vi "Exit Multi Frame Structure.vi"(0 "Diagram in":refnum<vi>, 5 "Outputs":refnum<vi>[][](array[refnum]), 11 "error in (no error)":errorcluster) -> (4 "Diagram out":refnum<vi>, 6 "Outputs":refnum<vi>[](array[refnum]), 15 "error out":errorcluster)   [LabVIEW 2015, in "Scripting.lvlib"]
doc: "Exits the Multi Frame Structure that owns <B>Diagram in</B>, supplying the structure's owning diagram at <B>Diagram out</B>."
uses:
  Scripting.lvlib
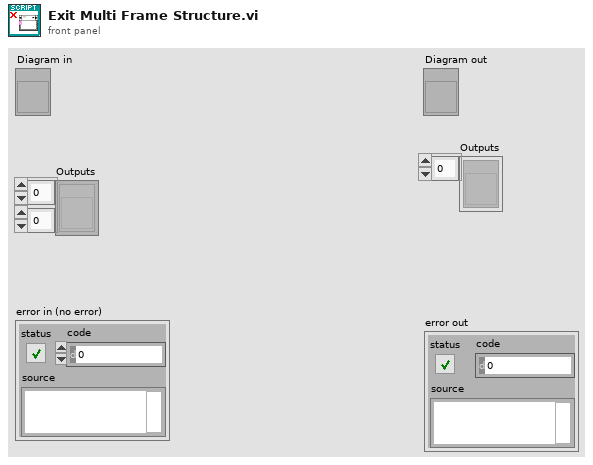
[diagram p1: front panel]
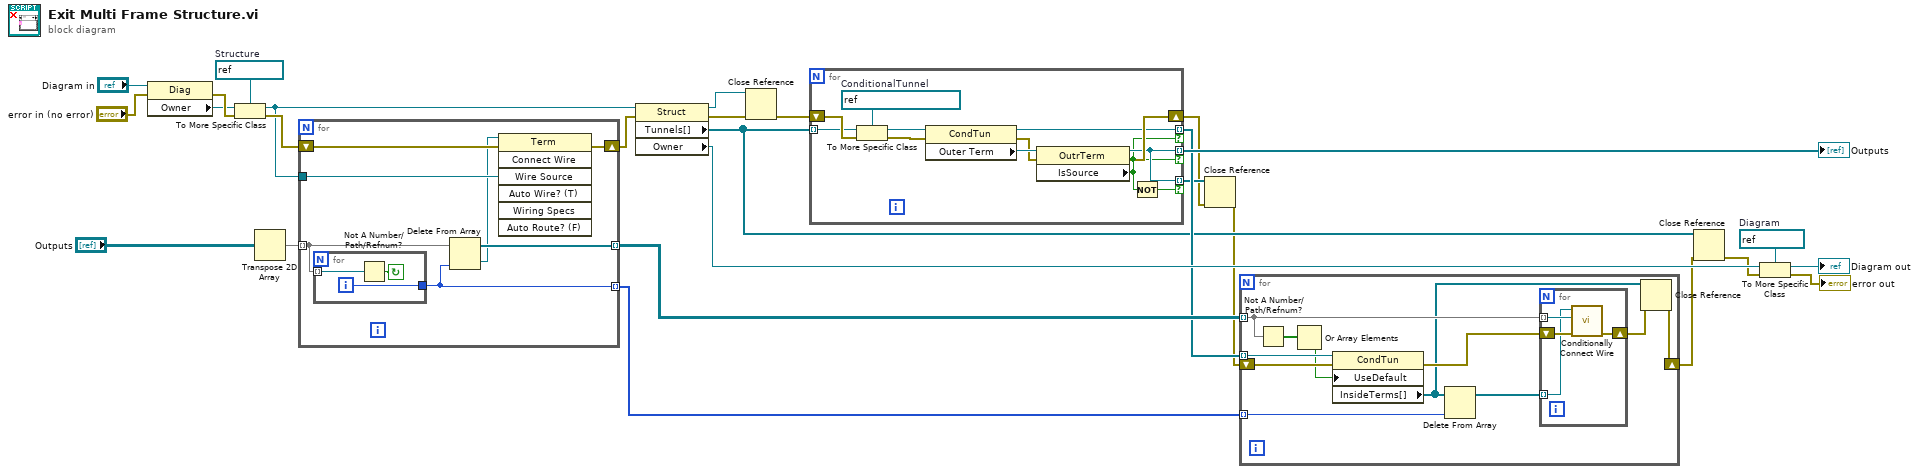
[diagram p0: block diagram]
diagram:
  w23 = refnum<vi> refnum  # Diagram
  w25 = refnum<vi> refnum  # Structure
  n1 = property class="Diag"(reference="Diagram in", error in="error in (no error)") -> (error out=w26:errorcluster, "Owner"=w24:refnum<vi>)  [unwired: 1 out]
  n2 = To More Specific Class(target class=w25, reference=w24, error in=w26) -> (specific class reference=w21:refnum<vi>, error out=w27:errorcluster)
  n3 = Transpose 2D Array(2D array="Outputs") -> (transposed array=w13:refnum<vi>[][])
  n4 = for {
    tunnel: w21 -> [w33]
    shift-right: [w32] -> w20
    shift-left: w27 -> [w34]
    tunnel: w13 -> [w28] mode=indexing
    tunnel: [w31] -> w19 mode=indexing
    tunnel: [w29] -> w9 mode=indexing
    n5 = for {
      tunnel: w28 -> [w35] mode=indexing
      tunnel: [w36] -> w29
      i -> [w36]
      stop <- w37 continue-if-true
      n6 = Not A Number/Path/Refnum?(number/path/refnum=w35) -> (NaN/Path/Refnum?=w37:bool)
    }
    n7 = Delete From Array(array=w28, index=w29) -> (deleted portion=w30:refnum<vi>, array with subset deleted=w31:refnum<vi>[])  [unwired: 1 in]
    n8 = invoke class="Term" method="Connect Wire"(reference=w30, error in=w34, "Wire Source"=w33) -> (error out=w32:errorcluster)  [unwired: 4 in, 6 out]
  }
  n9 = property class="Struct"(reference=w21, error in=w20) -> (reference out=w7:refnum<vi>, error out=w12:errorcluster, "Tunnels[]"=w6:refnum<vi>[], "Owner"=w22:refnum<vi>)
  n10 = Close Reference(reference=w7, error in (no error)=w12) -> (error out=w8:errorcluster)
  n11 = for {
    tunnel: w6 -> [w43] mode=indexing
    tunnel: [w40] -> w15 mode=indexing if=w38
    shift-right: [w46] -> w2
    shift-left: w8 -> [w49]
    tunnel: [w45] -> w14 mode=indexing if=w38
    tunnel: [w40] -> w3 mode=indexing if=w39
    w41 = refnum<vi> refnum  # ConditionalTunnel
    n12 = To More Specific Class(target class=w41, reference=w43, error in=w49) -> (specific class reference=w42:refnum<vi>, error out=w44:errorcluster)
    n13 = property class="CondTun"(reference=w42, error in=w44) -> (reference out=w45:refnum<vi>, error out=w47:errorcluster, "Outer Term"=w48:refnum<vi>)
    n14 = property class="OutrTerm"(reference=w48, error in=w47) -> (reference out=w40:refnum<vi>, error out=w46:errorcluster, "IsSource"=w38:bool)
    n15 = Not(x=w38) -> (.not. x?=w39:bool)
  }
  "Outputs" <- w15
  n16 = Close Reference(reference=w3, error in (no error)=w2) -> (error out=w1:errorcluster)
  n17 = for {
    tunnel: w14 -> [w60] mode=indexing
    shift-right: [w51] -> w5
    shift-left: w1 -> [w59]
    tunnel: w19 -> [w56] mode=indexing
    tunnel: w9 -> [w53] mode=indexing
    n18 = Not A Number/Path/Refnum?(number/path/refnum=w56) -> (NaN/Path/Refnum?=w55:bool[])
    n19 = Or Array Elements(Boolean array=w55) -> (logical OR=w54:bool)
    n20 = property class="CondTun"(reference=w60, error in=w59, "UseDefault"=w54) -> (error out=w58:errorcluster, "InsideTerms[]"=w50:refnum<vi>[])  [unwired: 1 out]
    n21 = Delete From Array(array=w50, index=w53) -> (array with subset deleted=w57:refnum<vi>[])  [unwired: 1 in, 1 out]
    n22 = for {
      shift-right: [w63] -> w52
      shift-left: w58 -> [w64]
      tunnel: w57 -> [w61] mode=indexing
      tunnel: w56 -> [w62] mode=indexing
      n23 = call "Conditionally Connect Wire.vi"("error in (no error)"=w64, "Wire Source"=w62, "Terminal in"=w61) -> ("error out"=w63:errorcluster)  [unwired: 7 in, 1 out]
    }
    n24 = Close Reference(reference=w50, error in (no error)=w52) -> (error out=w51:errorcluster)
  }
  n25 = Close Reference(reference=w6, error in (no error)=w5) -> (error out=w4:errorcluster)
  n26 = To More Specific Class(target class=w23, reference=w22, error in=w4) -> (specific class reference=→"Diagram out":refnum<vi>, error out=→"error out":errorcluster)
